vi "ATF Storage-Datalog Display NS creater.vi"(9 "Data FIFO Ref":T1) -> ()   [LabVIEW 2022 SP3]
uses:
  RT Controls/ATF Storage-Data FIFO.ctl
  RT Controls/ATF Storage-DiplayPC comm ctrl.ctl
  <vilib>/dex/Stream Element Allocation Mode.ctl
  ATF Storage-RT_Global_R.vi
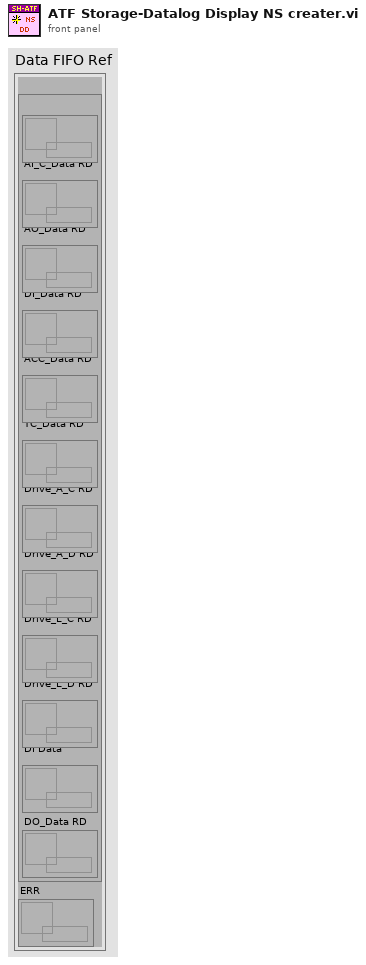
[diagram p1: front panel]
types:
  T1 = typedef "ATF Storage-Data FIFO.ctl" = cluster{"RD":cluster{"AI_V_Data RD":refnum<queue>, "AI_C_Data RD":refnum<queue>, "AO_Data RD":refnum<queue>, "DI_Data RD":refnum<queue>, "ACC_Data RD":refnum<queue>, "TC_Data RD":refnum<queue>, "Drive_A_C RD":refnum<queue>, "Drive_A_D RD":refnum<queue>, "Drive_L_C RD":refnum<queue>, "Drive_L_D RD":refnum<queue>, "DI Data":refnum<queue>, "DO_Data RD":refnum<queue>}, "ERR":refnum<queue>}
  T2 = typedef "ATF Storage-DiplayPC comm ctrl.ctl" = enum16{"Initialize", "Listen for UI Writer", "Send RT Data"}
  T3 = typedef "Stream Element Allocation Mode.ctl" = u32
  T4 = cluster{"Start DAQ":bool, "Stop DAQ":bool, "RT Stop":bool, "RT Exit":bool, "Start Seq":bool}
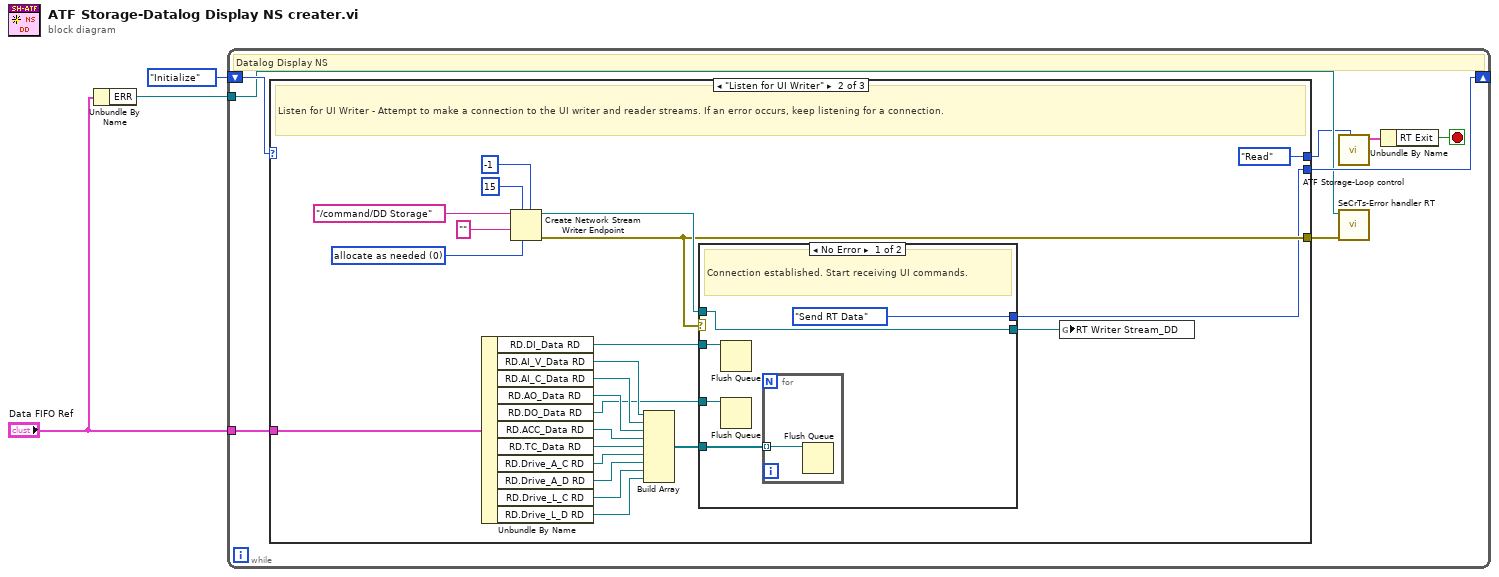
[diagram p0: block diagram]
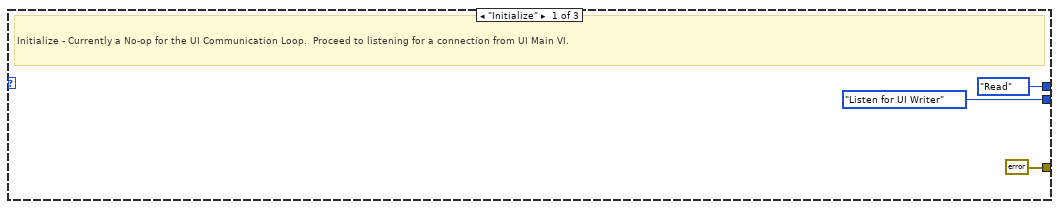
[diagram p2: hidden frame]
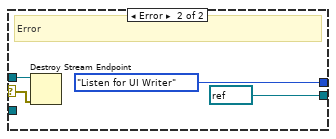
[diagram p3: hidden frame]
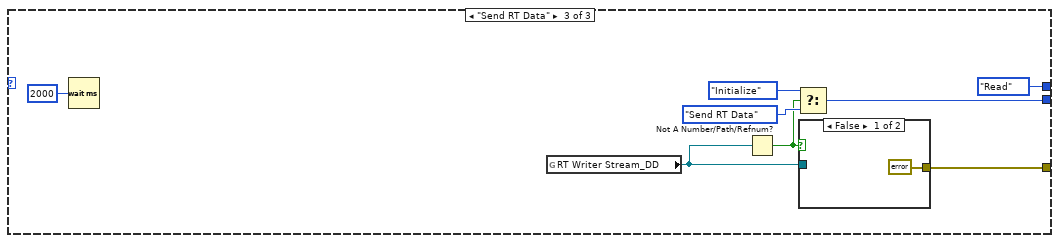
[diagram p4: hidden frame]
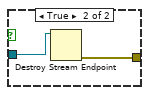
[diagram p5: hidden frame]
diagram:
  n1 = Unbundle By Name("Data FIFO Ref") -> ("ERR"=w1:refnum<queue>)
  n2 = while {
    shift-right: [w11] -> _
    shift-left: ATF_Storage-DiplayPC_comm_ctrl."Initialize" -> [w10]
    tunnel: "Data FIFO Ref" -> [w9]
    tunnel: w1 -> [w6]
    stop <- w7 stop-if-true
    # "Datalog Display NS"
    n3 = case shown="\"Listen for UI Writer\"" w10 {
      tunnel: [errorcluster {"status"=FALSE, "code"=0, "source"=""} ("error IO") w36 w49] -> w5
      tunnel: [ATF_Storage-DiplayPC_comm_ctrl."Listen for UI Writer" w35 w54] -> w11
      tunnel: w9 -> [_ w32 _]
      tunnel: [enum16{"Init", "Write", "Read"}."Read" ("Action") enum16{"Init", "Write", "Read"}."Read" ("Action") enum16{"Init", "Write", "Read"}."Read" ("Action")] -> w4
      frame "Initialize" {
        # "Initialize - Currently a No-op for the UI Communication Loop.  Proceed to listening for a connection from UI Main VI."
      }
      frame "Listen for UI Writer" {
        w17 = T3 0 items=["allocate as needed", "pre-allocate"] ("element allocation mode")
        # "Listen for UI Writer - Attempt to make a connection to the UI writer and reader streams. If an error occurs, keep listening for a connection."
        n4 = Unbundle By Name(w32) -> ("RD.DI_Data RD"=w19:refnum<queue>, "RD.AI_V_Data RD"=w29:refnum<queue>, "RD.AI_C_Data RD"=w28:refnum<queue>, "RD.AO_Data RD"=w27:refnum<queue>, "RD.DO_Data RD"=w16:refnum<queue>, "RD.ACC_Data RD"=w26:refnum<queue>, "RD.TC_Data RD"=w25:refnum<queue>, "RD.Drive_A_C RD"=w24:refnum<queue>, "RD.Drive_A_D RD"=w23:refnum<queue>, "RD.Drive_L_C RD"=w22:refnum<queue>, "RD.Drive_L_D RD"=w21:refnum<queue>)
        n5 = Create Network Stream Writer Endpoint(5:-1 ("timeout in ms (-1)"), 6:w17, 7:15 ("writer buffer size"), 9:"" ("reader url"), 11:"/command/DD Storage" ("reader url")) -> (0:w36:errorcluster, 3:w37:refnum<k21>)  [unwired: 2 in]
        n6 = Build Array(w29, w28, w27, w26, w25, w24, w23, w22, w21) -> (w20:refnum<queue>[])
        n7 = case shown="No Error" w36 {
          selector: w36 -> [_ w45]
          tunnel: w37 -> [w41 w47]
          tunnel: [ATF_Storage-DiplayPC_comm_ctrl."Send RT Data" ATF_Storage-DiplayPC_comm_ctrl."Listen for UI Writer"] -> w35
          tunnel: [w41 refnum<k21> refnum ("reader url")] -> w30
          tunnel: w20 -> [w40 _]
          tunnel: w19 -> [w39 _]
          tunnel: w16 -> [w38 _]
          frame No Error {
            # "Connection established. Start receiving UI commands."
            n8 = Flush Queue(queue=w39) -> ()  [unwired: 1 in, 3 out]
            n9 = Flush Queue(queue=w38) -> ()  [unwired: 1 in, 3 out]
            n10 = for {
              tunnel: w40 -> [w43] mode=indexing
              n11 = Flush Queue(queue=w43) -> ()  [unwired: 1 in, 3 out]
            }
          }
          frame Error {
            # "Error"
            n12 = Destroy Stream Endpoint(8:w45, 11:w47) -> ()  [unwired: 1 out]
          }
        }
        n13 = global write "ATF Storage-RT_Global_R.vi" "RT Writer Stream_DD"(w30) -> ()
      }
      frame "Send RT Data" {
        n14 = Wait (ms)(milliseconds to wait=u32 2000) -> ()  [unwired: 1 out]
        n15 = global read "ATF Storage-RT_Global_R.vi" "RT Writer Stream_DD"() -> (w50:refnum<k21>)
        n16 = Not A Number/Path/Refnum?(number/path/refnum=w50) -> (NaN/Path/Refnum?=w51:bool)
        n17 = Select(t=ATF_Storage-DiplayPC_comm_ctrl."Initialize", s=w51, f=ATF_Storage-DiplayPC_comm_ctrl."Send RT Data") -> (s? t:f=w54:T2)
        n18 = case shown="False" w51 {
          tunnel: w50 -> [_ w58]
          tunnel: [errorcluster {"status"=FALSE, "code"=0, "source"=""} ("error out") w57] -> w49
          frame False {
          }
          frame True {
            n19 = Destroy Stream Endpoint(11:w58) -> (0:w57:errorcluster)  [unwired: 1 in]
          }
        }
      }
    }
    n20 = call "ATF Storage-Loop control.vi"("Action"=w4) -> ("Loop Control out"=w8:T4)  [unwired: 9 in, 1 out]
    n21 = call "SeCrTs-Error handler RT.vi"("error in"=w5, "Message Queue"=w6) -> ()  [unwired: 8 in, 2 out]
    n22 = Unbundle By Name(w8) -> ("RT Exit"=w7:bool)
  }
